vi "FlatToRichw4lvgrpc_ToClient.vi"(5 "OutputClusterType":T1, 11 "InputCluster":T2) -> (3 "OutputCluster":T1)   [LabVIEW 2019, in "Generated_server.lvlib"]
uses:
  Generated_server.lvlib
  w4lvgrpc_ToClient_payload/w4lvgrpc_ToClient_payload.lvclass
  w4lvgrpc_ToClient.ctl
  w4lvgrpc_Msg_ToClient_9_Flat.ctl
  w4lvgrpc_Msg_ToClient_8_Flat.ctl
  w4lvgrpc_Msg_ToClient_7_Flat.ctl
  w4lvgrpc_Msg_ToClient_6_Flat.ctl
  w4lvgrpc_Msg_ToClient_5_Flat.ctl
  w4lvgrpc_Msg_ToClient_4_Flat.ctl
  w4lvgrpc_State.ctl
  w4lvgrpc_Msg_ToClient_3_Flat.ctl
  w4lvgrpc_Msg_ToClient_2_Flat.ctl
  w4lvgrpc_Msg_ToClient_1_Flat.ctl
  w4lvgrpc_ToClient_Flat.ctl
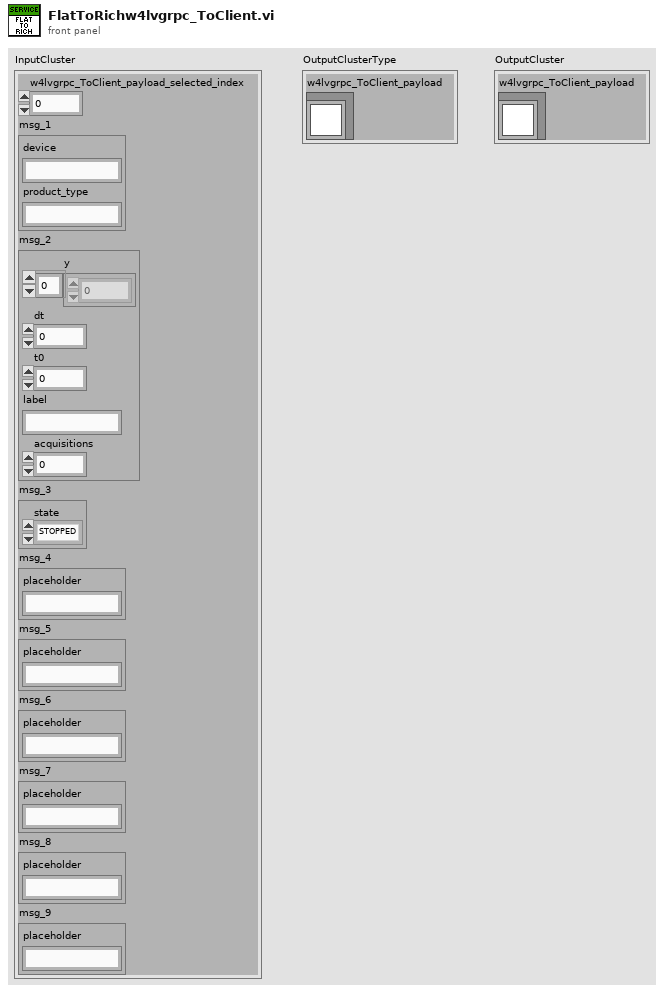
[diagram p1: front panel]
types:
  T1 = typedef "Generated_server.lvlib/w4lvgrpc_ToClient.ctl" = cluster{"w4lvgrpc_ToClient_payload":refnum<class "w4lvgrpc_ToClient_payload.lvclass">}
  T2 = typedef "Generated_server.lvlib/w4lvgrpc_ToClient_Flat.ctl" = cluster{"w4lvgrpc_ToClient_payload_selected_index":i32, "msg_1":T3, "msg_2":T4, "msg_3":T5, "msg_4":T7, "msg_5":T8, "msg_6":T9, "msg_7":T10, "msg_8":T11, "msg_9":T12}
  T3 = typedef "Generated_server.lvlib/w4lvgrpc_Msg_ToClient_1_Flat.ctl" = cluster{"device":string, "product_type":string}
  T4 = typedef "Generated_server.lvlib/w4lvgrpc_Msg_ToClient_2_Flat.ctl" = cluster{"y":dbl[], "dt":dbl, "t0":dbl, "label":string, "acquisitions":i32}
  T5 = typedef "Generated_server.lvlib/w4lvgrpc_Msg_ToClient_3_Flat.ctl" = cluster{"state":T6}
  T6 = typedef "Generated_server.lvlib/w4lvgrpc_State.ctl" = enum32{"STOPPED", "RUNNING", "ERROR"}
  T7 = typedef "Generated_server.lvlib/w4lvgrpc_Msg_ToClient_4_Flat.ctl" = cluster{"placeholder":string}
  T8 = typedef "Generated_server.lvlib/w4lvgrpc_Msg_ToClient_5_Flat.ctl" = cluster{"placeholder":string}
  T9 = typedef "Generated_server.lvlib/w4lvgrpc_Msg_ToClient_6_Flat.ctl" = cluster{"placeholder":string}
  T10 = typedef "Generated_server.lvlib/w4lvgrpc_Msg_ToClient_7_Flat.ctl" = cluster{"placeholder":string}
  T11 = typedef "Generated_server.lvlib/w4lvgrpc_Msg_ToClient_8_Flat.ctl" = cluster{"placeholder":string}
  T12 = typedef "Generated_server.lvlib/w4lvgrpc_Msg_ToClient_9_Flat.ctl" = cluster{"placeholder":string}
  T13 = typedef "Generated_server.lvlib/w4lvgrpc_Msg_ToClient_1.ctl" = cluster{"device":string, "product_type":string}
  T14 = typedef "Generated_server.lvlib/w4lvgrpc_Msg_ToClient_2.ctl" = cluster{"y":dbl[], "dt":dbl, "t0":dbl, "label":string, "acquisitions":i32}
  T15 = typedef "Generated_server.lvlib/w4lvgrpc_Msg_ToClient_3.ctl" = cluster{"state":T6}
  T16 = typedef "Generated_server.lvlib/w4lvgrpc_Msg_ToClient_4.ctl" = cluster{"placeholder":string}
  T17 = typedef "Generated_server.lvlib/w4lvgrpc_Msg_ToClient_5.ctl" = cluster{"placeholder":string}
  T18 = typedef "Generated_server.lvlib/w4lvgrpc_Msg_ToClient_6.ctl" = cluster{"placeholder":string}
  T19 = typedef "Generated_server.lvlib/w4lvgrpc_Msg_ToClient_7.ctl" = cluster{"placeholder":string}
  T20 = typedef "Generated_server.lvlib/w4lvgrpc_Msg_ToClient_8.ctl" = cluster{"placeholder":string}
  T21 = typedef "Generated_server.lvlib/w4lvgrpc_Msg_ToClient_9.ctl" = cluster{"placeholder":string}
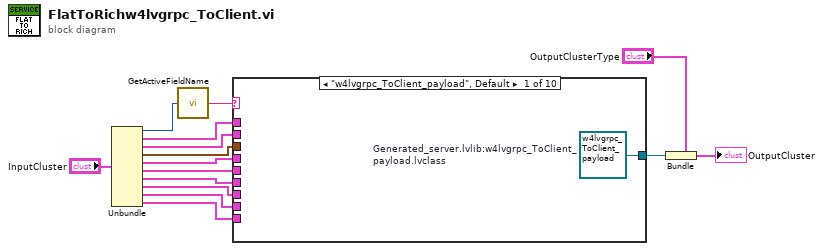
[diagram p0: block diagram]
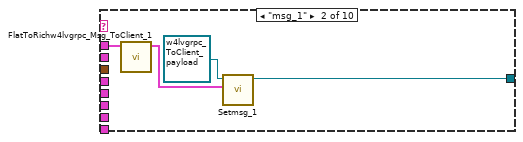
[diagram p2: hidden frame]
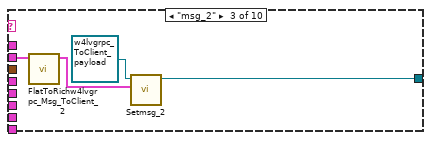
[diagram p3: hidden frame]
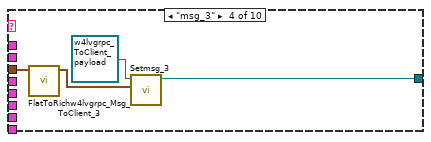
[diagram p4: hidden frame]
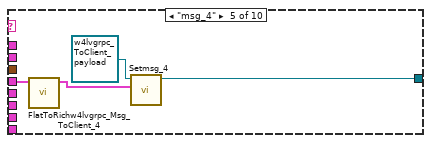
[diagram p5: hidden frame]
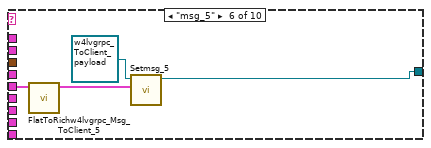
[diagram p6: hidden frame]
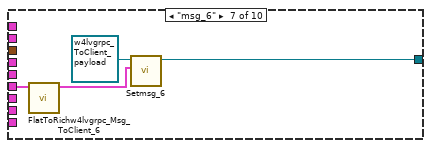
[diagram p7: hidden frame]
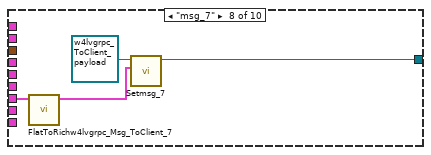
[diagram p8: hidden frame]
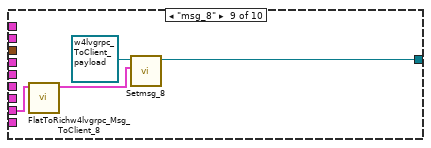
[diagram p9: hidden frame]
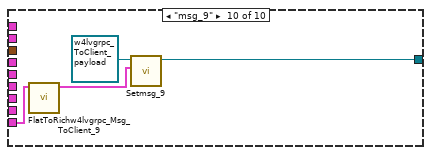
[diagram p10: hidden frame]
diagram:
  n1 = Unbundle "Unbundle"("InputCluster") -> ("w4lvgrpc_ToClient_payload_selected_index"=w12:i32, "msg_1"=w9:T3, "msg_2"=w8:T4, "msg_3"=w7:T5, "msg_4"=w6:T7, "msg_5"=w5:T8, "msg_6"=w4:T9, "msg_7"=w3:T10, "msg_8"=w2:T11, "msg_9"=w1:T12)
  n2 = call "GetActiveFieldName.vi"("protobuf index"=w12) -> ("oneof field name"=w11:string)
  n3 = case "w4lvgrpc_ToClient_payload" shown="\"w4lvgrpc_ToClient_payload\", Default" w11 {
    tunnel: [w16 w18 w22 w26 w30 w34 w38 w42 w46 w50] -> w10
    tunnel: w9 -> [_ w20 _ _ _ _ _ _ _ _]
    tunnel: w8 -> [_ _ w24 _ _ _ _ _ _ _]
    tunnel: w7 -> [_ _ _ w28 _ _ _ _ _ _]
    tunnel: w6 -> [_ _ _ _ w32 _ _ _ _ _]
    tunnel: w5 -> [_ _ _ _ _ w36 _ _ _ _]
    tunnel: w4 -> [_ _ _ _ _ _ w40 _ _ _]
    tunnel: w3 -> [_ _ _ _ _ _ _ w44 _ _]
    tunnel: w2 -> [_ _ _ _ _ _ _ _ w48 _]
    tunnel: w1 -> [_ _ _ _ _ _ _ _ _ w52]
    frame "w4lvgrpc_ToClient_payload", Default {
      w16 = refnum<class "w4lvgrpc_ToClient_payload.lvclass"> refnum  # Generated_server.lvlib:w4lvgrpc_ToClient_payload.lvclass
    }
    frame "msg_1" {
      n4 = call "FlatToRichw4lvgrpc_Msg_ToClient_1.vi"("InputCluster"=w20) -> ("OutputCluster"=w19:T13)  [unwired: 10 in]
      n5 = call "Setmsg_1.vi"("Set_Val"=w19, "OneOfTemplate in"=refnum<class "w4lvgrpc_ToClient_payload.lvclass"> refnum) -> ("OneOfTemplate out"=w18:refnum<class "w4lvgrpc_ToClient_payload.lvclass">)  [unwired: 8 in, 1 out]
    }
    frame "msg_2" {
      n6 = call "FlatToRichw4lvgrpc_Msg_ToClient_2.vi"("InputCluster"=w24) -> ("OutputCluster"=w23:T14)  [unwired: 10 in]
      n7 = call "Setmsg_2.vi"("Set_Val"=w23, "OneOfTemplate in"=refnum<class "w4lvgrpc_ToClient_payload.lvclass"> refnum) -> ("OneOfTemplate out"=w22:refnum<class "w4lvgrpc_ToClient_payload.lvclass">)  [unwired: 8 in, 1 out]
    }
    frame "msg_3" {
      n8 = call "FlatToRichw4lvgrpc_Msg_ToClient_3.vi"("InputCluster"=w28) -> ("OutputCluster"=w27:T15)  [unwired: 10 in]
      n9 = call "Setmsg_3.vi"("Set_Val"=w27, "OneOfTemplate in"=refnum<class "w4lvgrpc_ToClient_payload.lvclass"> refnum) -> ("OneOfTemplate out"=w26:refnum<class "w4lvgrpc_ToClient_payload.lvclass">)  [unwired: 8 in, 1 out]
    }
    frame "msg_4" {
      n10 = call "FlatToRichw4lvgrpc_Msg_ToClient_4.vi"("InputCluster"=w32) -> ("OutputCluster"=w31:T16)  [unwired: 10 in]
      n11 = call "Setmsg_4.vi"("Set_Val"=w31, "OneOfTemplate in"=refnum<class "w4lvgrpc_ToClient_payload.lvclass"> refnum) -> ("OneOfTemplate out"=w30:refnum<class "w4lvgrpc_ToClient_payload.lvclass">)  [unwired: 8 in, 1 out]
    }
    frame "msg_5" {
      n12 = call "FlatToRichw4lvgrpc_Msg_ToClient_5.vi"("InputCluster"=w36) -> ("OutputCluster"=w35:T17)  [unwired: 10 in]
      n13 = call "Setmsg_5.vi"("Set_Val"=w35, "OneOfTemplate in"=refnum<class "w4lvgrpc_ToClient_payload.lvclass"> refnum) -> ("OneOfTemplate out"=w34:refnum<class "w4lvgrpc_ToClient_payload.lvclass">)  [unwired: 8 in, 1 out]
    }
    frame "msg_6" {
      n14 = call "FlatToRichw4lvgrpc_Msg_ToClient_6.vi"("InputCluster"=w40) -> ("OutputCluster"=w39:T18)  [unwired: 10 in]
      n15 = call "Setmsg_6.vi"("Set_Val"=w39, "OneOfTemplate in"=refnum<class "w4lvgrpc_ToClient_payload.lvclass"> refnum) -> ("OneOfTemplate out"=w38:refnum<class "w4lvgrpc_ToClient_payload.lvclass">)  [unwired: 8 in, 1 out]
    }
    frame "msg_7" {
      n16 = call "FlatToRichw4lvgrpc_Msg_ToClient_7.vi"("InputCluster"=w44) -> ("OutputCluster"=w43:T19)  [unwired: 10 in]
      n17 = call "Setmsg_7.vi"("Set_Val"=w43, "OneOfTemplate in"=refnum<class "w4lvgrpc_ToClient_payload.lvclass"> refnum) -> ("OneOfTemplate out"=w42:refnum<class "w4lvgrpc_ToClient_payload.lvclass">)  [unwired: 8 in, 1 out]
    }
    frame "msg_8" {
      n18 = call "FlatToRichw4lvgrpc_Msg_ToClient_8.vi"("InputCluster"=w48) -> ("OutputCluster"=w47:T20)  [unwired: 10 in]
      n19 = call "Setmsg_8.vi"("Set_Val"=w47, "OneOfTemplate in"=refnum<class "w4lvgrpc_ToClient_payload.lvclass"> refnum) -> ("OneOfTemplate out"=w46:refnum<class "w4lvgrpc_ToClient_payload.lvclass">)  [unwired: 8 in, 1 out]
    }
    frame "msg_9" {
      n20 = call "FlatToRichw4lvgrpc_Msg_ToClient_9.vi"("InputCluster"=w52) -> ("OutputCluster"=w51:T21)  [unwired: 10 in]
      n21 = call "Setmsg_9.vi"("Set_Val"=w51, "OneOfTemplate in"=refnum<class "w4lvgrpc_ToClient_payload.lvclass"> refnum) -> ("OneOfTemplate out"=w50:refnum<class "w4lvgrpc_ToClient_payload.lvclass">)  [unwired: 8 in, 1 out]
    }
  }
  n22 = Bundle "Bundle"(cluster="OutputClusterType", "w4lvgrpc_ToClient_payload"=w10) -> (→"OutputCluster":T1)
